vi "VI Eliminador 0.vi"(11 "Array in":u32[](array[numeric])) -> (3 "Array out":u32[](array[numeric]))   [LabVIEW 2017]
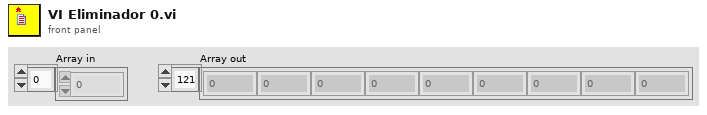
[diagram p1: front panel]
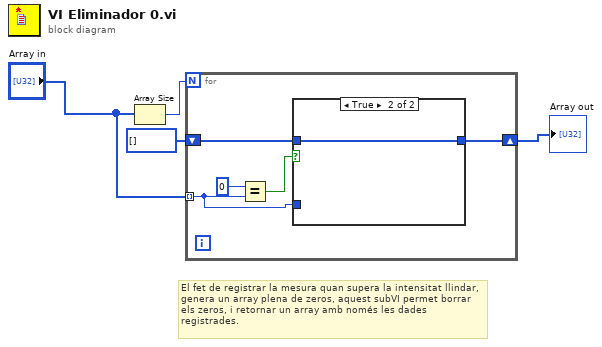
[diagram p0: block diagram]
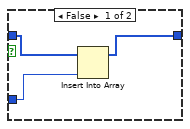
[diagram p2: hidden frame]
diagram:
  # "El fet de registrar la mesura quan supera la intensitat llindar, genera un array plena de zeros, aquest subVI permet borrar els zeros, i retornar un array amb només les dades registrades."
  n1 = Array Size(array="Array in") -> (size(s)=w1:i32)
  n2 = for {
    N: w1 -> [_]
    tunnel: "Array in" -> [w7] mode=indexing
    shift-right: [w5] -> w4
    shift-left: u32[] [] -> [w6]
    n3 = Equal?(x=u32 0, y=w7) -> (x = y?=w8:bool)
    n4 = case shown="True" w8 {
      tunnel: w7 -> [w12 _]
      tunnel: w6 -> [w11 w13]
      tunnel: [w10 w13] -> w5
      frame False {
        n5 = Insert Into Array(array=w11, new element=w12) -> (w10:u32[])  [unwired: 1 in]
      }
      frame True {
      }
    }
  }
  "Array out" <- w4
